vi "Profile Control.vi"(6 "Control Mode":T1, 8 "error in (no error)":errorcluster, 10 "Profile Number":u32=1 min=1 max=40 step=1, 11 "F4T in":refnum<class "F4T.lvclass">) -> (0 "error out":errorcluster, 3 "F4T out":refnum<class "F4T.lvclass">)   [LabVIEW 2018, in "F4T.lvlib" / "F4T.lvclass"]
doc: "This Override is used to Start, Pause, Resume or Stop a Profile.\n\nProfile Number is Mandatory with the <START> Mode, unused for the rest of the modes."
uses:
  F4T.lvclass
  PPLs/Temp Chamber/Parent/Temp Chamber.lvlibp/Custom Controls/Control Mode.ctl
  Custom Controls/Command Data.ctl
  PPLs/Temp Chamber/Parent/Temp Chamber.lvlibp/Temp Chamber.lvclass
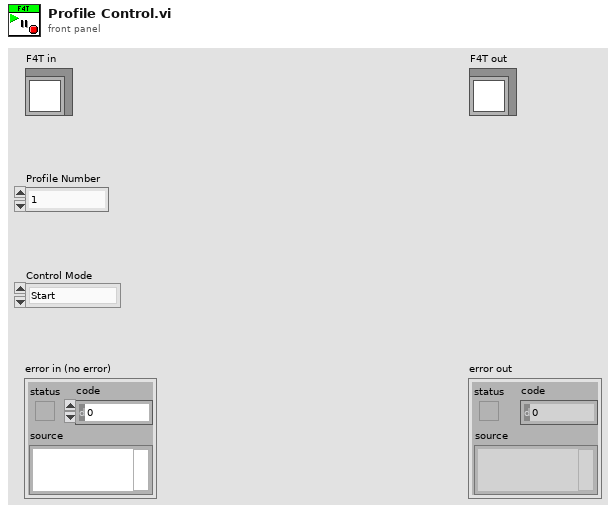
[diagram p1: front panel]
types:
  T1 = typedef "Temp Chamber.lvlibp/Temp Chamber.lvclass/Control Mode.ctl" = enum16{"Start", "Pause", "Resume", "Stop"}
  T2 = typedef "F4T.lvlib/F4T.lvclass/Command Data.ctl" = cluster{"ParameterID":u32, "InstanceId":u32, "Value":string}
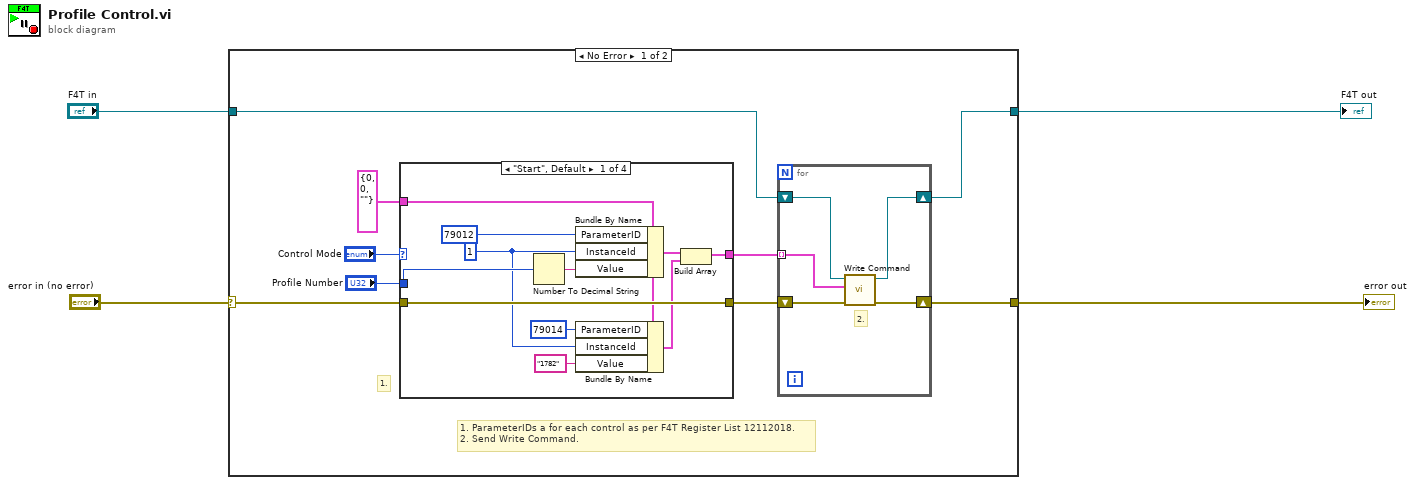
[diagram p0: block diagram]
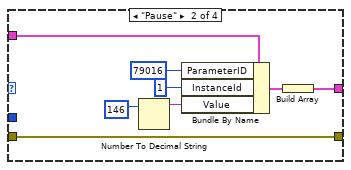
[diagram p2: hidden frame]
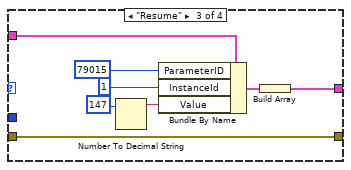
[diagram p3: hidden frame]
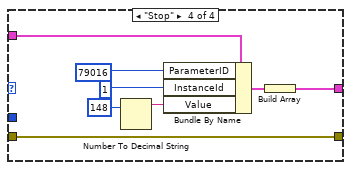
[diagram p4: hidden frame]
diagram:
  n1 = case shown="No Error" "error in (no error)" {
    selector: "error in (no error)" -> [w11 w55]
    tunnel: [w13 w55] -> w3
    tunnel: [w12 w54] -> w2
    tunnel: "F4T in" -> [w10 w54]
    frame No Error {
      # "1."
      # "1. ParameterIDs a for each control as per F4T Register List 12112018.\n2. Send Write Command."
      n2 = case shown="\"Start\", Default" "Control Mode" {
        tunnel: w11 -> [w29 w37 w45 w53]
        tunnel: [w29 w37 w45 w53] -> w8
        tunnel: "Profile Number" -> [w26 _ _ _]
        tunnel: T2 {"ParameterID"=0, "InstanceId"=0, "Value"=""} ("Command Data") -> [w25 w31 w42 w47]
        tunnel: [w19 w30 w38 w46] -> w5
        frame "Start", Default {
          w24 = u32 1 ("InstanceId")
          n3 = Number To Decimal String(number=w26) -> (decimal integer string=w28:string)  [unwired: 1 in]
          n4 = Bundle By Name(cluster=w25, "ParameterID"=u32 79012, "InstanceId"=w24, "Value"=w28) -> (w21:T2)
          n5 = Bundle By Name(cluster=w25, "ParameterID"=u32 79014, "InstanceId"=w24, "Value"="1782") -> (w20:T2)
          n6 = Build Array(w21, w20) -> (w19:T2[])
        }
        frame "Pause" {
          n7 = Number To Decimal String(number=u32 146 ("Profile Number")) -> (decimal integer string=w33:string)  [unwired: 1 in]
          n8 = Bundle By Name(cluster=w31, "ParameterID"=u32 79016, "InstanceId"=u32 1, "Value"=w33) -> (w32:T2)
          n9 = Build Array(w32) -> (w30:T2[])
        }
        frame "Resume" {
          n10 = Number To Decimal String(number=u32 147 ("Profile Number")) -> (decimal integer string=w44:string)  [unwired: 1 in]
          n11 = Bundle By Name(cluster=w42, "ParameterID"=u32 79015, "InstanceId"=u32 1, "Value"=w44) -> (w43:T2)
          n12 = Build Array(w43) -> (w38:T2[])
        }
        frame "Stop" {
          n13 = Number To Decimal String(number=u32 148 ("Profile Number")) -> (decimal integer string=w52:string)  [unwired: 1 in]
          n14 = Bundle By Name(cluster=w47, "ParameterID"=u32 79016, "InstanceId"=u32 1, "Value"=w52) -> (w51:T2)
          n15 = Build Array(w51) -> (w46:T2[])
        }
      }
      n16 = for {
        shift-right: [w17] -> w12
        shift-left: w10 -> [w16]
        shift-right: [w18] -> w13
        shift-left: w8 -> [w15]
        tunnel: w5 -> [w14] mode=indexing
        # "2."
        n17 = call "Write Command.vi"("error in (no error)"=w15, "Command Data"=w14, "F4T in"=w16) -> ("error out"=w18:errorcluster, "F4T out"=w17:refnum<class "F4T.lvclass">)  [unwired: 7 in]
      }
    }
    frame Error {
    }
  }
  "error out" <- w3
  "F4T out" <- w2
